vi "Quadrature.vi"   [LabVIEW 2017, in "NI_AALPro.lvlib"]
doc: "Performs numerical integration using adaptive quadrature approach. You must manually select the polymorphic instance to use."
uses:
  <vilib>/Analysis/NI_AALPro.lvlib
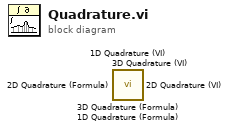
[diagram p0: block diagram]
diagram:
  n1 = call <vilib>:"3D Quadrature (Formula).vi"() -> ()  [unwired: 10 in, 2 out]
  n2 = call <vilib>:"3D Quadrature (VI).vi"() -> ()  [unwired: 10 in, 2 out]
  n3 = call <vilib>:"2D Quadrature (Formula).vi"() -> ()  [unwired: 10 in, 2 out]
  n4 = call <vilib>:"2D Quadrature (VI).vi"() -> ()  [unwired: 10 in, 2 out]
  n5 = call <vilib>:"1D Quadrature (Formula).vi"() -> ()  [unwired: 10 in, 2 out]
  n6 = call <vilib>:"1D Quadrature (VI).vi"() -> ()  [unwired: 10 in, 2 out]
